vi "Remote uService GUI.vi"(7 "Message Enqueuer":refnum<class "Common GUI v3.lvclass">, 10 "GUI VI":refnum<vi>, 11 "uService ID":string) -> ()   [LabVIEW 2026, in "TALOS.lvlib" / "Common GUI v3.lvlib"]
uses:
  Common GUI v3.lvlib
  Common GUI v3/Common GUI v3.lvclass
  C:/LabVIEW Code/TALOS/talos/Father of all uServices/Father of all uServices/Father of all uServices.lvclass
  Remote uService GUI.ctl
  Common GUI v3/Common GUI v3 Consumer Case Selector.ctl
  Father of all uServices/Father of all uServices Messages/Consumer Msg/Consumer Msg.lvclass/Consumer Msg.ctl
  Ancestor/Ancestor/Ancestor.lvclass/Ancestor.ctl
  Father of all uServices/Father of all uServices Messages/Consumer Msg/Send Consumer.vi
  Support VIs/Substitute Error.vi
  Support VIs/Generate Error.vi
  FGV/Error Memory/Get Error Description.vi
  Support VIs/Get PC name.vi
  Ancestor/Ancestor/Read ID.vi
  Support VIs/Get Class Name.vi
  <vilib>/Utility/error.llb/Clear Errors.vi
  FGV/Error Memory/Error Memory Core.vi
  <vilib>/AdvancedString/Delimited String to 1D String Array.vi
  <vilib>/AdvancedString/Delimited String to 1D String Array (string).vi
  Support VIs/Circus Root Path.vi
  FGV/Error Memory/Error Crt Lvl checker.vi
  FGV/Error Memory/Error Memory Core.vi/40c8088d-b597-4017-91af-faa98e00292e.vi
  FGV/Error Memory/Error Memory Core.vi/d4a3ab98-063c-4e44-b43d-fbdcfe6c2be2.vi
  Father of all uServices/Father of all uServices/Father of all uServices.lvclass
  C:/LabVIEW Code/TALOS/builds/Actor Framework PPL/Actor Framework.lvlibp/1abvi3w/vi.lib/ActorFramework/Actor/Actor.lvclass
  builds/Actor Framework PPL/Actor Framework.lvlibp/1abvi3w/vi.lib/ActorFramework/Actor/Read Self Enqueuer.vi
  <userlib>/_OpenG.lib/lvdata/lvdata.llb/Get Strings from Enum__ogtk.vi
  builds/Actor Framework PPL/Actor Framework.lvlibp/1abvi3w/vi.lib/ActorFramework/Message Enqueuer/Enqueue.vi
  Support VIs/Global Memory.vi
  <vilib>/Utility/LVClass/Get LV Class Name.vi
  Support VIs/Is in Packed Library.vi
  Support VIs/TALOS Root path.vi
  Support VIs/Read CSV worksheet.vi
  Support VIs/Global Constants.vi
  <vilib>/Utility/error.llb/General Error Handler.vi
  Support VIs/Error Log.vi
  Father of all uServices/Father of all uServices Messages/Consumer Msg/Consumer Msg.lvclass
  Ancestor/Ancestor/Ancestor.lvclass
  <vilib>/Comparison/Equal/Equal Functor/Equal Functor.lvclass
panel:
  in  "STOP":bool
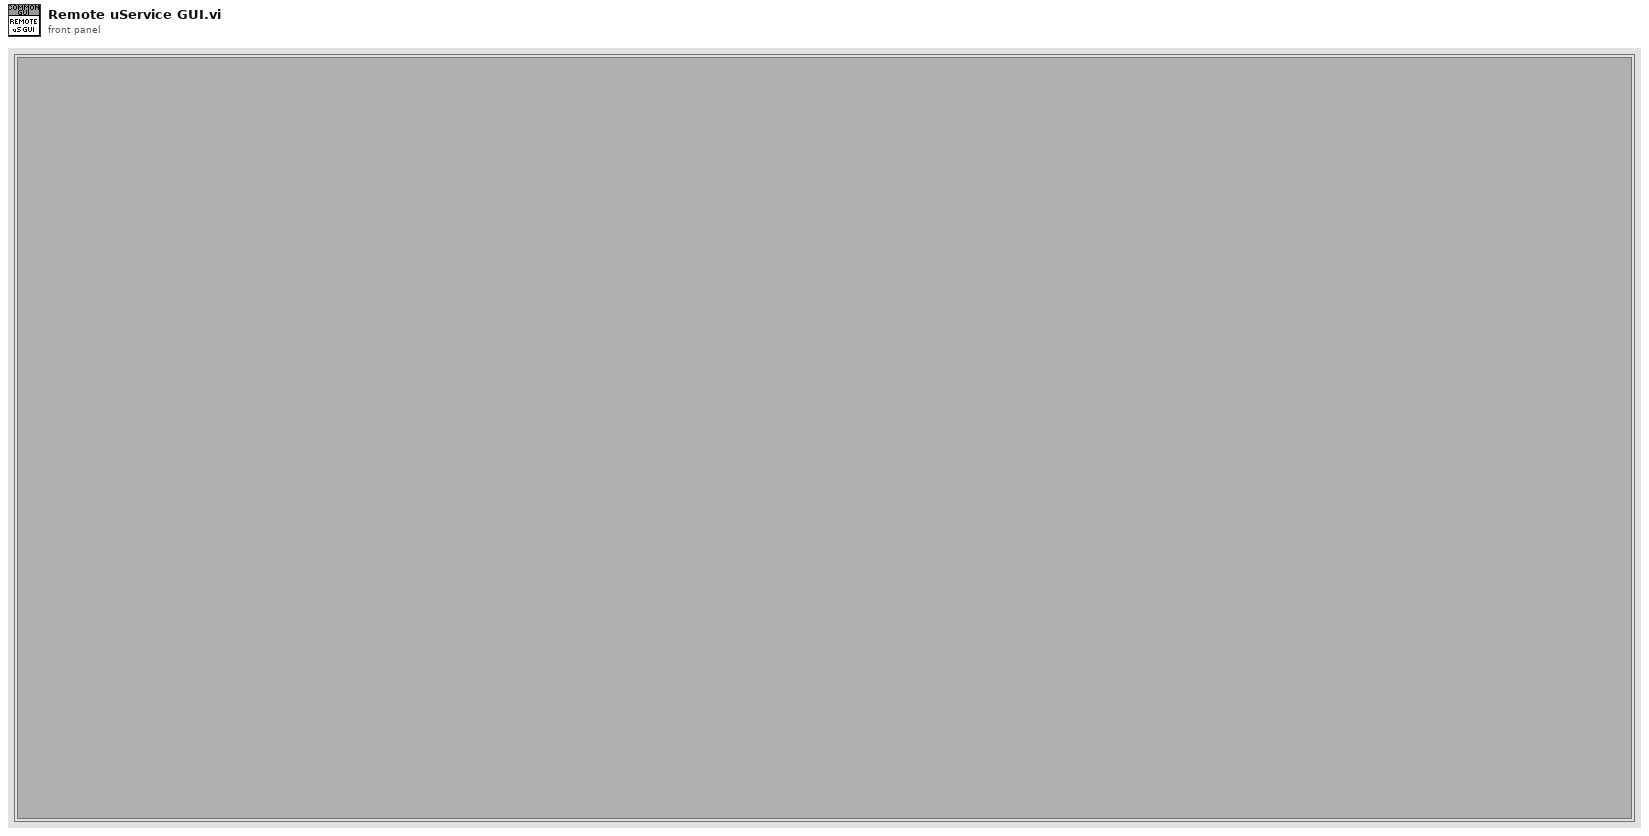
[diagram p1: front panel]
types:
  T1 = typedef "TALOS.lvlib/Common GUI v3.lvlib/Common GUI v3.lvclass/Common GUI v3 Consumer Case Selector.ctl" = enum16{"Update Guardians List", "Update ABORT LED", "Update Guardian ID", "Update Kasli Log", "Update Error Listbox", "Update Run Number", "Change Run LED color", "Update Run Status", "Run Stopped with Errors", "Reset Run LED", "Update Run Config", "Remote GUI"}
  T2 = typedef "TALOS.lvlib/Common GUI v3.lvlib/Remote uService GUI.ctl" = cluster{"Open/Close":bool, "uService ID":string}
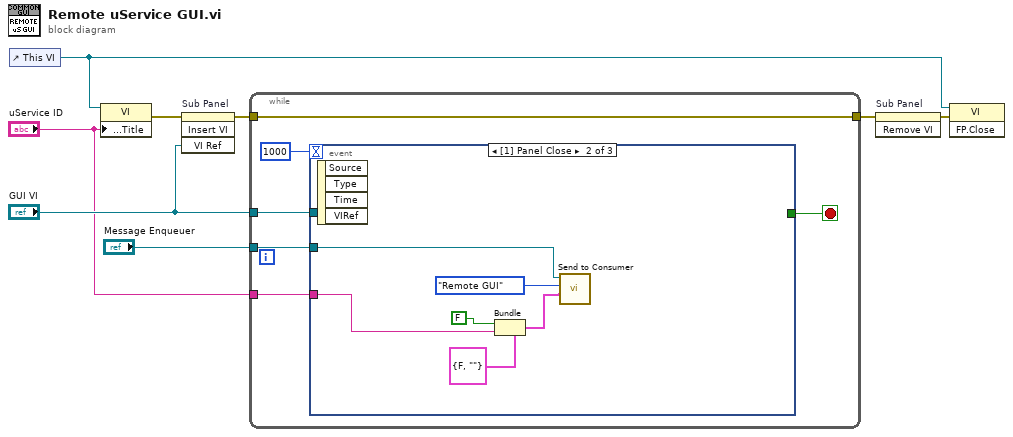
[diagram p0: block diagram]
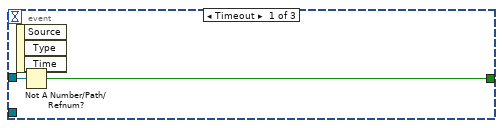
[diagram p2: hidden frame]
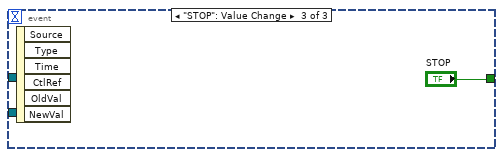
[diagram p3: hidden frame]
diagram:
  n1 = control-ref of="This VI"() -> (w5:refnum<vi>)
  n2 = property class="VI"(reference=w5, "Front Panel.Title"="uService ID") -> (error out=w3:errorcluster)  [unwired: 1 in, 1 out]
  n3 = invoke on="Sub Panel" class="SubPnl" method="Insert VI"(error in=w3, "VI Ref"="GUI VI") -> (error out=w8:errorcluster)  [unwired: 2 in, 3 out]
  n4 = while {
    tunnel: w8 -> [w11]
    tunnel: "GUI VI" -> [w14]
    tunnel: [w11] -> w6
    tunnel: "uService ID" -> [w10]
    tunnel: "Message Enqueuer" -> [w9]
    stop <- w13 stop-if-true
    n5 = event shown="[1] Panel Close" {
      selector: _ -> [_ _ _]
      dyn-events: _ -> [_ _ _]
      timeout: 1000 -> [_ _ _]
      tunnel: w14 -> [w16 _ _]
      tunnel: [w15 _ "STOP"] -> w13
      tunnel: w10 -> [_ w22 _]
      tunnel: w9 -> [_ w17 _]
      event Timeout {
        n6 = event-data() -> ()  [unwired: 1 in, 3 out]
        n7 = Not A Number/Path/Refnum?(number/path/refnum=w16) -> (NaN/Path/Refnum?=w15:bool)
      }
      event Panel Close {
        n8 = event-data() -> ()  [unwired: 1 in, 4 out]
        n9 = Bundle(cluster=T2 {"Open/Close"=FALSE, "uService ID"=""} ("Remote GUI"), "Open/Close"=FALSE, "uService ID"=w22) -> (w18:T2)
        n10 = call "Send to Consumer.vi"("Data"=w18, "Case ID"=Common_GUI_v3_Consumer_Case_Selector."Remote GUI" ("Template Internal v3 Consumer Case Selector"), "uService Template in"=w17) -> ()  [unwired: 7 in, 2 out]
      }
      event "STOP": Value Change {
        n11 = event-data() -> ()  [unwired: 1 in, 6 out]
      }
    }
  }
  n12 = invoke on="Sub Panel" class="SubPnl" method="Remove VI"(error in=w6) -> (error out=w4:errorcluster)  [unwired: 2 in, 2 out]
  n13 = invoke class="VI" method="FP.Close"(reference=w5, error in=w4) -> ()  [unwired: 1 in, 3 out]
